vi "aux-builder.vi"(10 "Proc Name":string, 11 "Cluster":T1={"Source"="Source ...", "SourceStatus"=FALSE, "Dest"="Auxiliary ...", "DestStatus"=FALSE, "Pulse"=0, "Period"=0, "Proc Name"=""} {"Period" format="Period [s]: %d"; "Pulse" format="Pulse [s]: %d"}) -> (3 "AUXI Flow":T2[](array[typedef]))   [LabVIEW 2024]
uses:
  controls/UiStepBuilder.ctl
  controls/type.step-builder.ctl
  controls/type.aux.ctl
  controls/UiDeviceSensorParams.ctl
  controls/UiDeviceSensorEquality.ctl
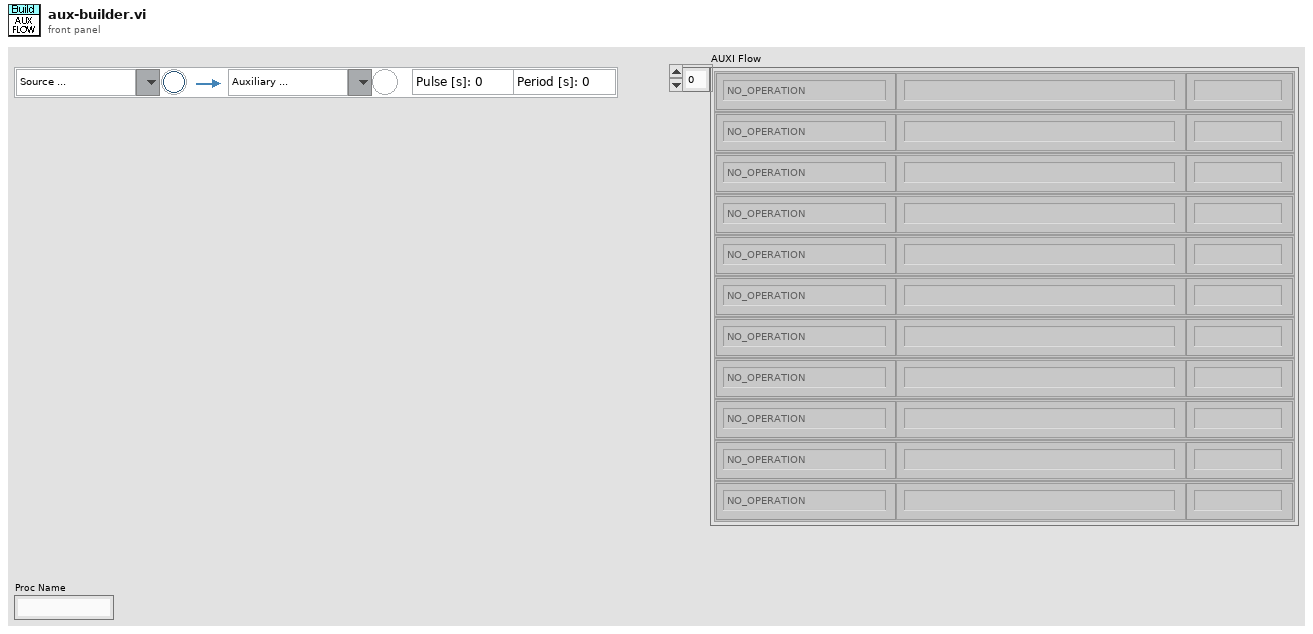
[diagram p1: front panel]
types:
  T1 = typedef "type.aux.ctl" = cluster{"Source":string, "SourceStatus":bool, "Dest":string, "DestStatus":bool, "Pulse":u16, "Period":u16, "Proc Name":string}
  T2 = typedef "UiStepBuilder.ctl" = cluster{"Step Function":T3, "ParamString":string, "Step Label":string}
  T3 = typedef "type.step-builder.ctl" = enum16{"NO_OPERATION", "DELAY-JUMP", "DELAY", "JUMP", "COMPLETE", "SCHEDULER", "IRR-CHECK", "UNIT-CHECK", "UNIT-SAMPLE", "UNIT-DOSE", "LOG-REPORT", "LOG-MESSAGE", "IO-READ", "IO-READ-MANY", "IO-WRITE", "IO-COMPARE-OUT", "IO-COMPARE-IN", "PROC-START", "PROC-STOP", "PROC-LOAD", "PROC-IS-COMPLETED", "RECORD-MOVE", "GET-RH", "GET-UV", "GET-WD", "GET-WS", "OCS-CHECK", "OCS-RECORD"}
  T4 = typedef "UiDeviceSensorEquality.ctl" = string
  T5 = typedef "UiDeviceSensorParams.ctl" = cluster{"Input":string, "Comparison":T4, "Setpoint":dbl}
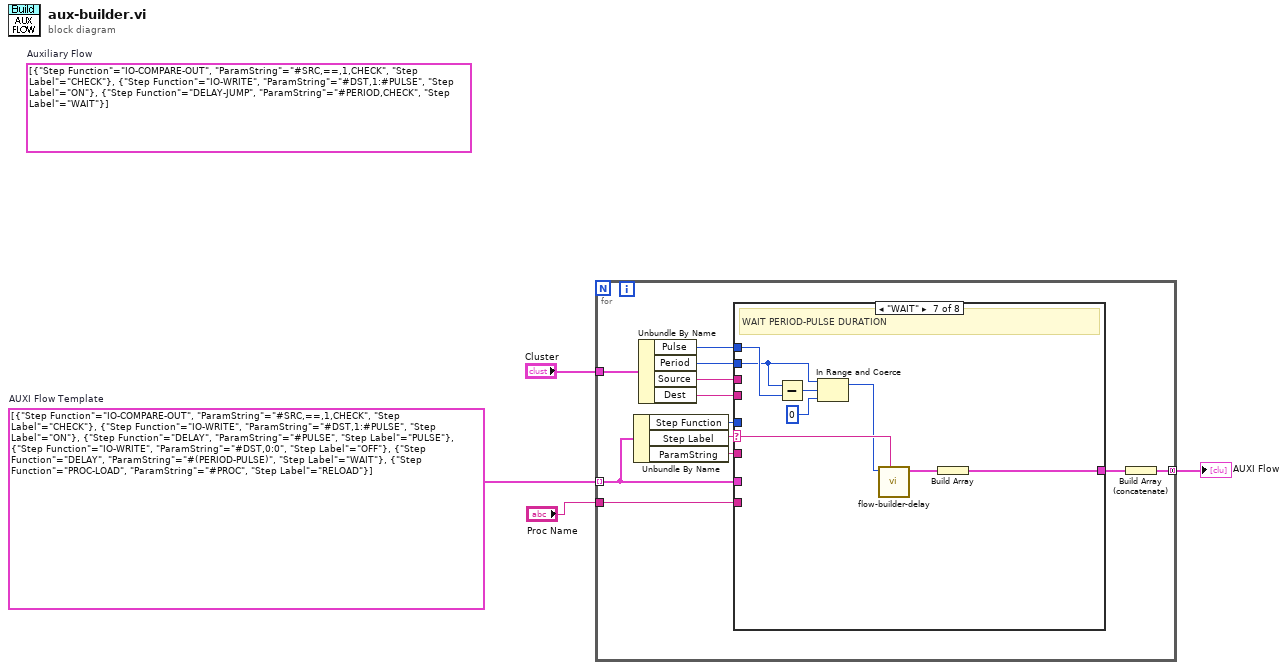
[diagram p0: block diagram]
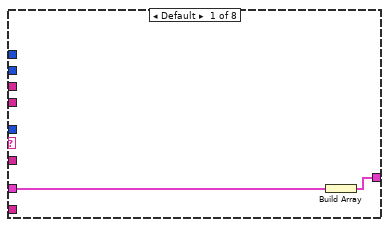
[diagram p2: hidden frame]
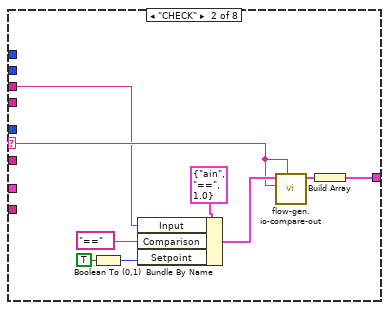
[diagram p3: hidden frame]
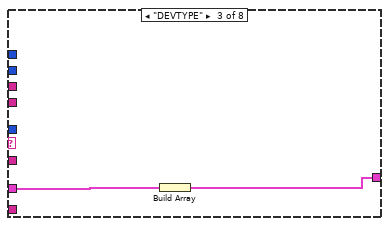
[diagram p4: hidden frame]
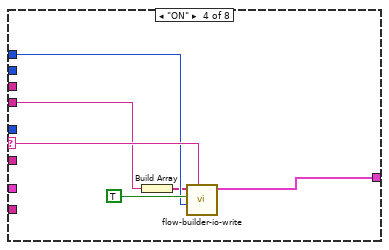
[diagram p5: hidden frame]
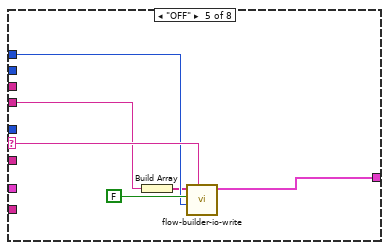
[diagram p6: hidden frame]
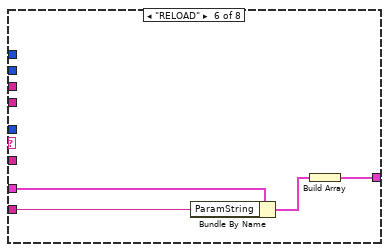
[diagram p7: hidden frame]
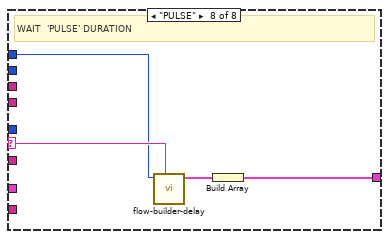
[diagram p8: hidden frame]
diagram:
  (unwired) T2[] [{"Step Function"=enum."IO-COMPARE-OUT", "ParamString"="#SRC,==,1,CHECK", "Step Label"="CHECK"}, {"Step Function"=enum."IO-WRITE", "ParamString"="#DST,1:#PULSE", "Step Label"="ON"}, {"Step Function"=enum."DELAY-JUMP", "ParamString"="#PERIOD,CHECK", "Step Label"="WAIT"}]  # Auxiliary Flow
  w4 = T2[] [{"Step Function"=enum."IO-COMPARE-OUT", "ParamString"="#SRC,==,1,CHECK", "Step Label"="CHECK"}, {"Step Function"=enum."IO-WRITE", "ParamString"="#DST,1:#PULSE", "Step Label"="ON"}, {"Step Function"=enum."DELAY", "ParamString"="#PULSE", "Step Label"="PULSE"}, {"Step Function"=enum."IO-WRITE", "ParamString"="#DST,0:0", "Step Label"="OFF"}, {"Step Function"=enum."DELAY", "ParamString"="#(PERIOD-PULSE)", "Step Label"="WAIT"}, {"Step Function"=enum."PROC-LOAD", "ParamString"="#PROC", "Step Label"="RELOAD"}]  # AUXI Flow Template
  n1 = for {
    tunnel: w4 -> [w15] mode=indexing
    tunnel: [w13] -> w3 mode=concatenating
    tunnel: "Cluster" -> [w10]
    tunnel: "Proc Name" -> [w5]
    n2 = Unbundle By Name(w15) -> ("Step Function"=w11:T3, "Step Label"=w16:string, "ParamString"=w12:string)
    n3 = Unbundle By Name(w10) -> ("Pulse"=w8:u16, "Period"=w6:u16, "Source"=w9:string, "Dest"=w7:string)
    n4 = case shown="\"WAIT\"" w16 {
      selector: w16 -> [_ w23 _ w34 w40 _ w52 w56]
      tunnel: w15 -> [w18 _ w28 _ _ w43 _ _]
      tunnel: [w17 w26 w29 w35 w41 w44 w51 w55] -> w14
      tunnel: w12 -> [_ _ _ _ _ _ _ _]
      tunnel: w11 -> [_ _ _ _ _ _ _ _]
      tunnel: w9 -> [_ w19 _ _ _ _ _ _]
      tunnel: w8 -> [_ _ _ w32 w38 _ w48 w54]
      tunnel: w7 -> [_ _ _ w31 w37 _ _ _]
      tunnel: w6 -> [_ _ _ _ _ _ w46 _]
      tunnel: w5 -> [_ _ _ _ _ w42 _ _]
      frame Default {
        n5 = Build Array(w18) -> (w17:T2[])
      }
      frame "CHECK" {
        n6 = Boolean To (0,1)(Boolean=TRUE) -> (0, 1=w20:i16)
        n7 = Bundle By Name(cluster=T5 {"Input"="ain", "Comparison"="==", "Setpoint"=1.0} ("UiDeviceParamsSensor"), "Input"=w19, "Comparison"=T4 "==", "Setpoint"=w20) -> (w24:T5)
        n8 = call "flow-gen.io-compare-out.vi"("Step Label"=w23, "stepPointer (False Cond.)"=w23, "Device Sensor Params"=w24) -> ("Step out"=w27:T2)  [unwired: 8 in]
        n9 = Build Array(w27) -> (w26:T2[])
      }
      frame "DEVTYPE" {
        n10 = Build Array(w28) -> (w29:T2[])
      }
      frame "ON" {
        n11 = Build Array(w31) -> (w30:string[])
        n12 = call "flow-builder-io-write.vi"("Step Name"=w34, "Digital Timeout"=w32, "Value in"=TRUE ("UiDeviceConstant"), "Dout+AUX"=w30) -> ("Flow out"=w35:T2[])  [unwired: 7 in]
      }
      frame "OFF" {
        n13 = Build Array(w37) -> (w36:string[])
        n14 = call "flow-builder-io-write.vi"("Step Name"=w40, "Digital Timeout"=w38, "Value in"=FALSE ("UiDeviceConstant"), "Dout+AUX"=w36) -> ("Flow out"=w41:T2[])  [unwired: 7 in]
      }
      frame "RELOAD" {
        n15 = Bundle By Name(cluster=w43, "ParamString"=w42) -> (w45:T2)
        n16 = Build Array(w45) -> (w44:T2[])
      }
      frame "WAIT" {
        # "WAIT PERIOD-PULSE DURATION"
        n17 = Subtract(x=w46, y=w48) -> (x-y=w50:u16)
        n18 = In Range and Coerce(upper limit=w46, x=w50, lower limit=u16 0) -> (coerced(x)=w49:u16)  [unwired: 1 out]
        n19 = call "flow-builder-delay.vi"("Step Label"=w52, "Delay [s]"=w49) -> ("Step Element"=w53:T2)  [unwired: 9 in]
        n20 = Build Array(w53) -> (w51:T2[])
      }
      frame "PULSE" {
        # "WAIT  'PULSE' DURATION"
        n21 = call "flow-builder-delay.vi"("Step Label"=w56, "Delay [s]"=w54) -> ("Step Element"=w57:T2)  [unwired: 9 in]
        n22 = Build Array(w57) -> (w55:T2[])
      }
    }
    n23 = Build Array (concatenate)(w14) -> (w13:T2[])
  }
  "AUXI Flow" <- w3
